vi "Coerce image size - SubVI.vi"(11 "Image Size":T1 {"V Bin" min=0.0; "H Bin" min=0.0 step=1.0}) -> (3 "Image Size 2":T1 {"V Bin" min=0.0; "H Bin" min=0.0 step=1.0})   [LabVIEW 2014]
uses:
  Camera Default Globals.vi
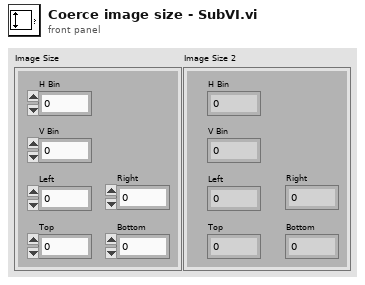
[diagram p1: front panel]
types:
  T1 = cluster{"H Bin":dbl, "V Bin":dbl, "Left":dbl, "Right":dbl, "Top":dbl, "Bottom":dbl}
  T2 = cluster{"H Bin":i32, "V Bin":i32, "Left":i32, "Top":i32, "Right":i32, "Bottom":i32}
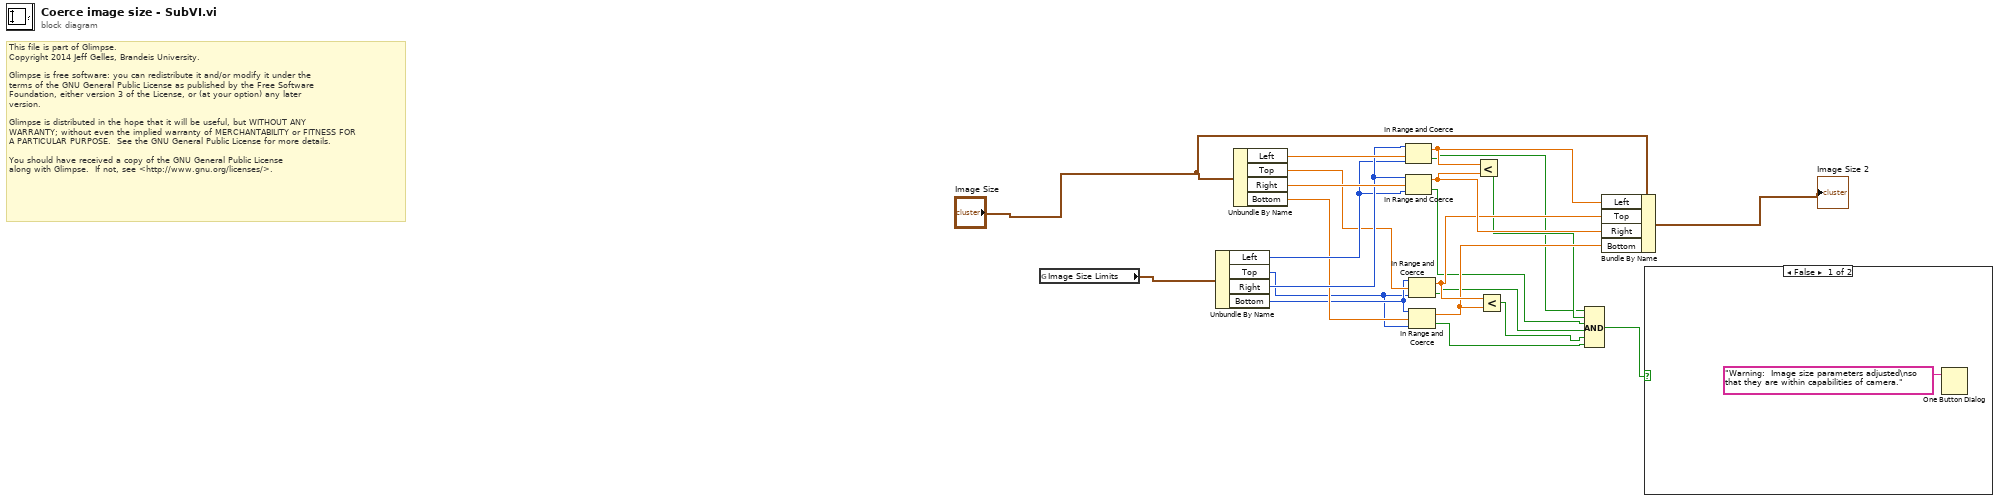
[diagram p0: block diagram]
diagram:
  # "This file is part of Glimpse. \nCopyright 2014 Jeff Gelles, Brandeis University.    \n\nGlimpse is free software: you can redistribute it and/or modify it under the \nterms of the GNU General Public License as published by the Free Software \nFoundation, either version 3 of the License, or (at your option) any later \nversion.\n\nGlimpse is distributed in the hope that it will be useful, but WITHOUT ANY \nWARRANTY; without even the implied warranty of MERCHANTABILITY or FITNESS FOR \nA PARTICULAR PURPOSE.  See the GNU General Public License for more details.\n\nYou should have received a copy of the GNU General Public License\nalong with Glimpse.  If not, see <http://www.gnu.org/licenses/>."
  n1 = global read "Camera Default Globals.vi" "Image Size Limits"() -> (w3:T2)
  n2 = Unbundle By Name(w3) -> ("Left"=w19:i32, "Top"=w13:i32, "Right"=w20:i32, "Bottom"=w14:i32)
  n3 = Unbundle By Name("Image Size") -> ("Left"=w22:dbl, "Top"=w16:dbl, "Right"=w21:dbl, "Bottom"=w15:dbl)
  n4 = In Range and Coerce(upper limit=w20, x=w22, lower limit=w19) -> (coerced(x)=w18:dbl, In Range?=w5:bool)
  n5 = In Range and Coerce(upper limit=w20, x=w21, lower limit=w19) -> (coerced(x)=w17:dbl, In Range?=w7:bool)
  n6 = In Range and Coerce(upper limit=w14, x=w16, lower limit=w13) -> (coerced(x)=w12:dbl, In Range?=w8:bool)
  n7 = In Range and Coerce(upper limit=w14, x=w15, lower limit=w13) -> (coerced(x)=w11:dbl, In Range?=w10:bool)
  n8 = Less?(x=w18, y=w17) -> (x < y?=w6:bool)
  n9 = Less?(x=w12, y=w11) -> (x < y?=w9:bool)
  n10 = Compound Arithmetic op=AND(w5, w6, w7, w8, w9, w10) -> (w4:bool)
  n11 = Bundle By Name(cluster="Image Size", "Left"=w18, "Top"=w12, "Right"=w17, "Bottom"=w11) -> (→"Image Size 2":T1)
  n12 = case shown="False" w4 {
    frame False {
      n13 = One Button Dialog(message="Warning:  Image size parameters adjusted\nso that they are within capabilities of camera.") -> ()  [unwired: 1 in, 1 out]
    }
    frame True {
    }
  }
